vi "Holo_link_test.vi"() -> ()   [LabVIEW 2023, in "holoTracker.lvlib"]
uses:
  holoTracker.lvlib
  <vilib>/Native 3D Graph/xcontrol/3DPC_SurfacePlot.xctl
panel:
  in  "minLenght":i32
  in  "stop":bool
  out "3D Graph":refnum<class "Base Datatype.lvclass">[](xcontrol)
  out "trajectorie":dbl[][](array[numeric])
  in  "feature_number":i32
  in  "memory":i32=1
  in  "searchRange":T1={"x_range(m)"=1e-06, "y_range(m)"=1e-06, "z__range(m)"=1e-06}
  out "size(s) 3":i32[](array[numeric])=[115588, 5]
  out "size(s) 2":i32[](array[numeric])=[115588, 5]
  out "size(s)":i32[](array[numeric])=[127033, 5]
  in  "voxel_size":i32=200
  out "return value":dbl[][](array[numeric])=[[1.0, 6.084467713662889e-06, 2.7942323868046515e-05, 5.448419528875093e-07, 370.0], [1.0, 0.0001626674929866, 3.476842903182842e-05, 2.303367864442407e-06, 5232.0], [1.0, 2.1535443011089228e-05, 4.458006515051238e-05, 8.414190233452246e-06, 11468.0], [1.0, 0.0001715506368782, 4.228565376251936e-05, 5.818839099447359e-07, 292.0], [1.0, 6.632606528000906e-05, 4.749142681248486e-05, 2.467622152835247e-06, 5073.0], [1.0, 0.0001096990090445, 4.7724013711558655e-05, 1.2655297041419544e-06, 662.0], [1.0, 0.0001106120907934, 5.094841617392376e-05, 1.1342979632900096e-05, 7273.0], [1.0, 0.0001622637646505, 5.3357507567852736e-05, 1.6849965049914315e-06, 1584.0], [1.0, 0.0001665420131757, 5.386502380133607e-05, 3.075804215768585e-06, 1222.0], [1.0, 8.49634816404432e-05, 6.137051968835294e-05, 1.222071750817122e-05, 70549.0], [1.0, 0.0001014012741507, 6.489593943115324e-05, 2.9947607345093274e-06, 2263.0], [1.0, 0.0001038984846672, 7.025278318906203e-05, 2.297732862643897e-06, 1479.0], [1.0, 2.920036604336929e-05, 7.49154351069592e-05, 5.151001005287981e-06, 16448.0], [1.0, 0.000173209249624, 7.902947982074693e-05, 1.5714367691543885e-05, 11413.0], [1.0, 7.337347051361576e-05, 8.688520756550133e-05, 3.910340183210792e-06, 6218.0], [1.0, 7.923282100819051e-05, 9.101555770030244e-05, 3.967892610035051e-07, 410.0], [1.0, 6.708591536153108e-05, 9.130484977504238e-05, 3.468035458809027e-07, 397.0], [1.0, 8.80229999893345e-05, 9.468459757044911e-05, 3.539114743489336e-07, 532.0], [1.0, 6.690550071652979e-05, 9.541779581923038e-05, 3.245157529363496e-07, 254.0], [1.0, 3.5517736250767484e-05, 0.0001058862326317, 8.118919367916533e-07, 1511.0], [1.0, 2.5897679734043777e-05, 0.0001085887779481, 4.002589776064269e-06, 1483.0], [1.0, 1.948640783666633e-05, 0.000112430032459, 1.9318811155244475e-06, 3982.0], [1.0, 0.0001211502676596, 0.0001132587276515, 3.043337073904695e-06, 6890.0], [1.0, 0.0001325271732639, 0.0001166411966551, 1.7197318811668083e-05, 73988.0], [1.0, 0.0001629522594157, 0.0001161332838819, 8.296568012156058e-06, 11009.0], [1.0, 0.0001552185276523, 0.0001186439185403, 2.3219217837322503e-06, 4923.0], [1.0, 0.0001647252065595, 0.0001183489002869, 5.199617589823902e-07, 138.0], [1.0, 0.0001584361452842, 0.0001295564579777, 7.808185387148114e-07, 283.0], [1.0, 0.000158121867571, 0.0001334999979007, 8.548132655050722e-07, 581.0], [1.0, 3.150296834064648e-05, 0.0001427773095201, 2.0931878680130467e-05, 79967.0], [1.0, 1.4578064110537524e-05, 0.0001393411366734, 2.624581156851491e-06, 8022.0], [1.0, 0.000163749748026, 0.0001381954352837, 2.6074342258652905e-06, 377.0], [1.0, 7.176306826295331e-05, 0.0001397340529365, 5.237333198238048e-07, 176.0], [1.0, 0.0001668064505793, 0.0001418412430211, 3.1187559557110944e-07, 278.0], [1.0, 3.841546276817098e-05, 0.0001423163776053, 5.334248953658971e-07, 504.0], [1.0, 1.4115883459453473e-05, 0.0001550480956211, 1.0434874639031476e-05, 87692.0], [1.0, 0.0001525868719909, 0.0001566513237776, 1.6795509509393014e-05, 68919.0], [1.0, 0.0001574417838128, 0.0001585431746207, 1.4897328526330966e-07, 268.0], [1.0, 0.0001097008935175, 0.0001609185419511, 1.1331389941915404e-06, 679.0], [1.0, 0.0001519046345492, 0.000164362398209, 8.700509397385758e-07, 957.0], [1.0, 6.392512295860797e-05, 0.0001700782158877, 4.624916982720606e-06, 26125.0], [1.0, 0.0001484176609665, 0.0001732027012621, 1.917527879413683e-05, 27440.0], [1.0, 0.0001644691219553, 0.0001723233290249, 1.057493022926792e-06, 577.0], [1.0, 0.0001374908024445, 0.0001755372941261, 4.3706279484467814e-07, 430.0], [1.0, 0.0001311707601416, 0.000170940067619, 5.035582489654189e-06, 178.0], [1.0, 0.0001576331706019, 0.0001583546836627, 5.210669314692495e-06, 183.0], [1.0, 6.659836799371988e-05, 9.181829227600248e-05, 1.0223350727756042e-05, 417.0], [1.0, 0.0001582865952514, 0.0001584510609973, 1.0296550499333534e-05, 358.0], [1.0, 0.0001036058311001, 6.883801688672975e-05, 2.46377367147943e-05, 8318.0], [1.0, 0.0001612922205822, 0.0001366157957818, 2.1547250071307644e-05, 4494.0], [1.0, 0.0001656974491197, 0.0001459676132071, 1.597193295310717e-05, 1142.0], [1.0, 8.80000734468922e-05, 9.563334606355056e-05, 1.5165374861680904e-05, 155.0], [1.0, 0.0001589283929206, 0.0001584299607202, 1.4875608030706644e-05, 120.0], [1.0, 0.0001571570464875, 0.0001176301957457, 1.8592216292745437e-05, 600.0], [1.0, 9.193427831633016e-05, 0.0001520802470622, 2.448859049763996e-05, 3245.0], [1.0, 0.000112866058771, 5.088346006232314e-05, 2.0907007638015784e-05, 381.0], [1.0, 0.0001208995527122, 5.201993917580694e-05, 2.5392644602106884e-05, 4814.0], [1.0, 3.008505518664606e-05, 0.0001077202978194, 3.3227548556169495e-05, 10644.0], [1.0, 2.0109948309254836e-05, 4.9624042731011286e-05, 2.6339754185755737e-05, 1424.0], [1.0, 0.0001608280290383, 0.0001719313731882, 2.710985245357733e-05, 351.0], [1.0, 8.62869928823784e-05, 5.857026553712785e-05, 3.342138370499015e-05, 4921.0], [1.0, 0.0001626797165954, 0.0001301088195759, 3.0994753615232185e-05, 2244.0], [1.0, 4.31185144407209e-05, 7.302458834601566e-05, 3.312131957500242e-05, 3267.0], [1.0, 0.0001629685575608, 0.0001367063232464, 3.083618139498867e-05, 960.0], [1.0, 0.0001743247848935, 0.0001414648722857, 3.15434044750873e-05, 632.0], [1.0, 0.0001613891945453, 0.0001737980928737, 4.036536120111123e-05, 5237.0], [1.0, 0.0001142588298534, 7.320034637814388e-05, 4.0086662920657545e-05, 7267.0], [1.0, 9.60408360697329e-05, 3.4551776479929686e-05, 3.70402995031327e-05, 3724.0], [1.0, 9.843446605373174e-06, 0.0001594874047441, 3.914430271834135e-05, 2684.0], [1.0, 0.0001547361607663, 5.664364653057419e-05, 3.706891948240809e-05, 2573.0], [1.0, 8.177998097380623e-05, 0.0001273784146178, 4.101425656699576e-05, 5968.0], [1.0, 0.0001532866881461, 9.97651950456202e-05, 4.03202539018821e-05, 2485.0], [1.0, 8.377496851608157e-05, 6.378004036378115e-05, 4.188828825135715e-05, 2325.0], [1.0, 6.149584078229964e-05, 6.080432285671122e-05, 4.78734727948904e-05, 12097.0], [1.0, 0.0001566413993714, 2.1062844098196365e-05, 5.120203059050255e-05, 9042.0], [1.0, 7.881547207944095e-05, 8.436228381469846e-05, 4.8256984882755205e-05, 6830.0], [1.0, 9.192600373353343e-06, 0.0001562820398248, 4.230014747008681e-05, 314.0], [1.0, 3.210443537682295e-05, 0.0001058917259797, 4.397206430439837e-05, 790.0], [1.0, 1.0259605431883757e-07, 0.0001552348112454, 4.410862675285898e-05, 124.0], [1.0, 0.0001500043581472, 3.777907477342524e-05, 4.75865017506294e-05, 5899.0], [1.0, 6.773022323613986e-05, 9.073886030819268e-05, 4.405568688525818e-05, 654.0], [1.0, 7.17540315235965e-05, 9.311777830589564e-05, 4.51631894975435e-05, 120.0], [1.0, 0.0001315168628934, 0.0001169017778011, 4.3997453758493066e-05, 275.0], [1.0, 8.366083784494549e-05, 9.656340262154116e-05, 5.384273754316382e-05, 8763.0], [1.0, 0.0001212393835885, 0.0001420576445525, 4.49199287686497e-05, 319.0], [1.0, 1.3556540352510638e-06, 0.0001552532194182, 4.509215796133503e-05, 175.0], [1.0, 0.0001683209993643, 0.000177976078703, 7.403743802569807e-05, 9925.0], [1.0, 7.289469067472965e-05, 7.800028834026307e-05, 5.28059717908036e-05, 2797.0], [1.0, 6.758869858458638e-05, 9.146620141109452e-05, 5.3512281738221645e-05, 1976.0], [1.0, 7.586500578327104e-05, 0.0001471474388381, 5.1613689720397815e-05, 1663.0], [1.0, 8.421528764301911e-05, 6.580434273928404e-05, 5.2117964514764026e-05, 1109.0], [1.0, 7.542532694060355e-05, 0.0001033193984767, 5.398859138949774e-05, 1832.0], [1.0, 3.501192622934468e-05, 0.0001395642757415, 5.483976929099299e-05, 5287.0], [1.0, 4.265514508006163e-05, 0.0001677416439633, 5.720457556890324e-05, 9416.0], [1.0, 7.38311791792512e-05, 0.0001008389881462, 5.14670173288323e-05, 145.0], [1.0, 7.137070497265086e-05, 9.350352047476918e-05, 5.3323659813031554e-05, 1723.0], [1.0, 0.0001614146895008, 9.723609400680289e-05, 5.891673208680004e-05, 4327.0], [1.0, 9.978431626223028e-05, 0.0001333983673248, 5.464206333272159e-05, 396.0], [1.0, 5.090175818622811e-06, 0.0001601206022314, 5.6050434068311006e-05, 894.0], [1.0, 9.459191642235965e-05, 6.544839561684057e-05, 7.306145562324673e-05, 29371.0], [1.0, 7.746577466605231e-05, 8.46039765747264e-05, 6.175429734867066e-05, 262.0], [1.0, 0.0001582324039191, 2.1445872334879823e-05, 6.363449210766703e-05, 870.0], [1.0, 3.7317844544304535e-05, 9.124814096139744e-05, 6.831272185081616e-05, 6541.0], [1.0, 1.784480809874367e-05, 0.0001019813425955, 6.767934974050149e-05, 2458.0], [1.0, 4.959088528266875e-06, 0.0001600535470061, 8.137130498653278e-05, 29776.0], [1.0, 3.297331932117231e-05, 0.0001390695833833, 6.774533540010452e-05, 1053.0], [1.0, 8.322825306095183e-05, 0.0001434805017197, 6.561006739502773e-05, 1939.0], [1.0, 0.0001370376121485, 9.71412009675987e-06, 6.492882675956935e-05, 291.0], [1.0, 0.0001772090326994, 3.539895624271594e-05, 6.882343586767092e-05, 3231.0], [1.0, 5.806188710266724e-05, 3.3593849366297945e-05, 6.884828326292336e-05, 2367.0], [1.0, 7.016197741904762e-06, 0.0001632697239983, 6.754777859896421e-05, 243.0], [1.0, 0.000170219267602, 0.0001663451548665, 7.293584349099547e-05, 4976.0], [1.0, 2.793159910652321e-05, 0.0001489773421781, 7.33017732272856e-05, 3999.0], [1.0, 0.0001163198103313, 6.302370456978679e-05, 7.591531903017312e-05, 3997.0], [1.0, 9.778481035027652e-05, 0.0001406495284754, 7.136896601878107e-05, 522.0], [1.0, 0.0001691433571977, 5.961917963759333e-07, 8.129586058203131e-05, 4070.0], [1.0, 1.4097173334448598e-05, 8.226431236835197e-05, 7.784627086948603e-05, 6167.0], [1.0, 2.436563590890728e-05, 1.974108090507798e-05, 8.088676258921623e-05, 7748.0], [1.0, 1.164888817584142e-05, 3.0726434488315135e-05, 8.314807928400114e-05, 3895.0], [1.0, 7.282009755726904e-05, 0.0001352824474452, 7.63883363106288e-05, 4002.0], [1.0, 0.0001400399924023, 0.0001319663715548, 8.391532901441678e-05, 8537.0], [1.0, 5.5921103921718895e-05, 0.000108788088255, 9.001097350846976e-05, 17549.0], [1.0, 0.000113057278213, 6.979489990044385e-05, 9.000674617709592e-05, 13550.0], [1.0, 0.0001127664218074, 9.079198207473382e-05, 8.478527161059901e-05, 8091.0], [1.0, 5.82017055421602e-05, 0.0001726192276692, 8.456128853140399e-05, 3833.0], [1.0, 1.0619457498250997e-05, 0.0001078733839676, 8.637746941531077e-05, 2405.0], [1.0, 2.520033740438521e-05, 0.000139325245982, 8.391139999730512e-05, 213.0], [1.0, 3.813329021795653e-05, 0.0001060482827597, 9.526589565211908e-05, 7139.0], [1.0, 0.0001007989849313, 7.21739706932567e-05, 9.082954784389584e-05, 1228.0], [1.0, 2.592455712147057e-05, 0.0001495852629886, 9.255921759177e-05, 200.0], [1.0, 4.128223008592613e-05, 4.959827856509946e-05, 9.645039244787768e-05, 6037.0], [1.0, 2.4412151105934757e-05, 0.0001384778734063, 9.155422594631092e-05, 365.0], [1.0, 5.305964077706449e-05, 0.0001283856399822, 9.582766506355256e-05, 4738.0], [1.0, 6.284587288973853e-05, 0.0001460118510294, 9.61513869697228e-05, 4087.0], [1.0, 2.5871122488752007e-05, 0.0001011573331197, 9.672308078734204e-05, 6301.0], [1.0, 4.819215610041283e-05, 9.018560376716778e-05, 9.685708209872246e-05, 1391.0], [1.0, 9.311481699114664e-05, 5.986811811453663e-05, 9.666049299994484e-05, 1440.0], [1.0, 8.8207729277201e-05, 3.934404958272353e-05, 9.83873542281799e-05, 2241.0], [1.0, 9.761466935742646e-05, 6.031811426510103e-05, 9.7536867542658e-05, 136.0], [1.0, 4.385911233839579e-05, 0.0001729830109979, 9.793794743018223e-05, 170.0], [1.0, 5.7778866903390735e-05, 0.0001088508433895, 9.875508112600072e-05, 357.0]]
  in  "Frame":i32=1
  out "error out":errorcluster
  out "Features":dbl[][](array[numeric])
  in  "holo Feature file":path=path "C:/TRAVAIL/developpement/imagesHolo/1000im_manip3/HOLO_2023_06_28_11_56_10.csv"
  in  "PythonVer":string="3.10" caption="Python version"
  in  "Python/Environnement\npath":path
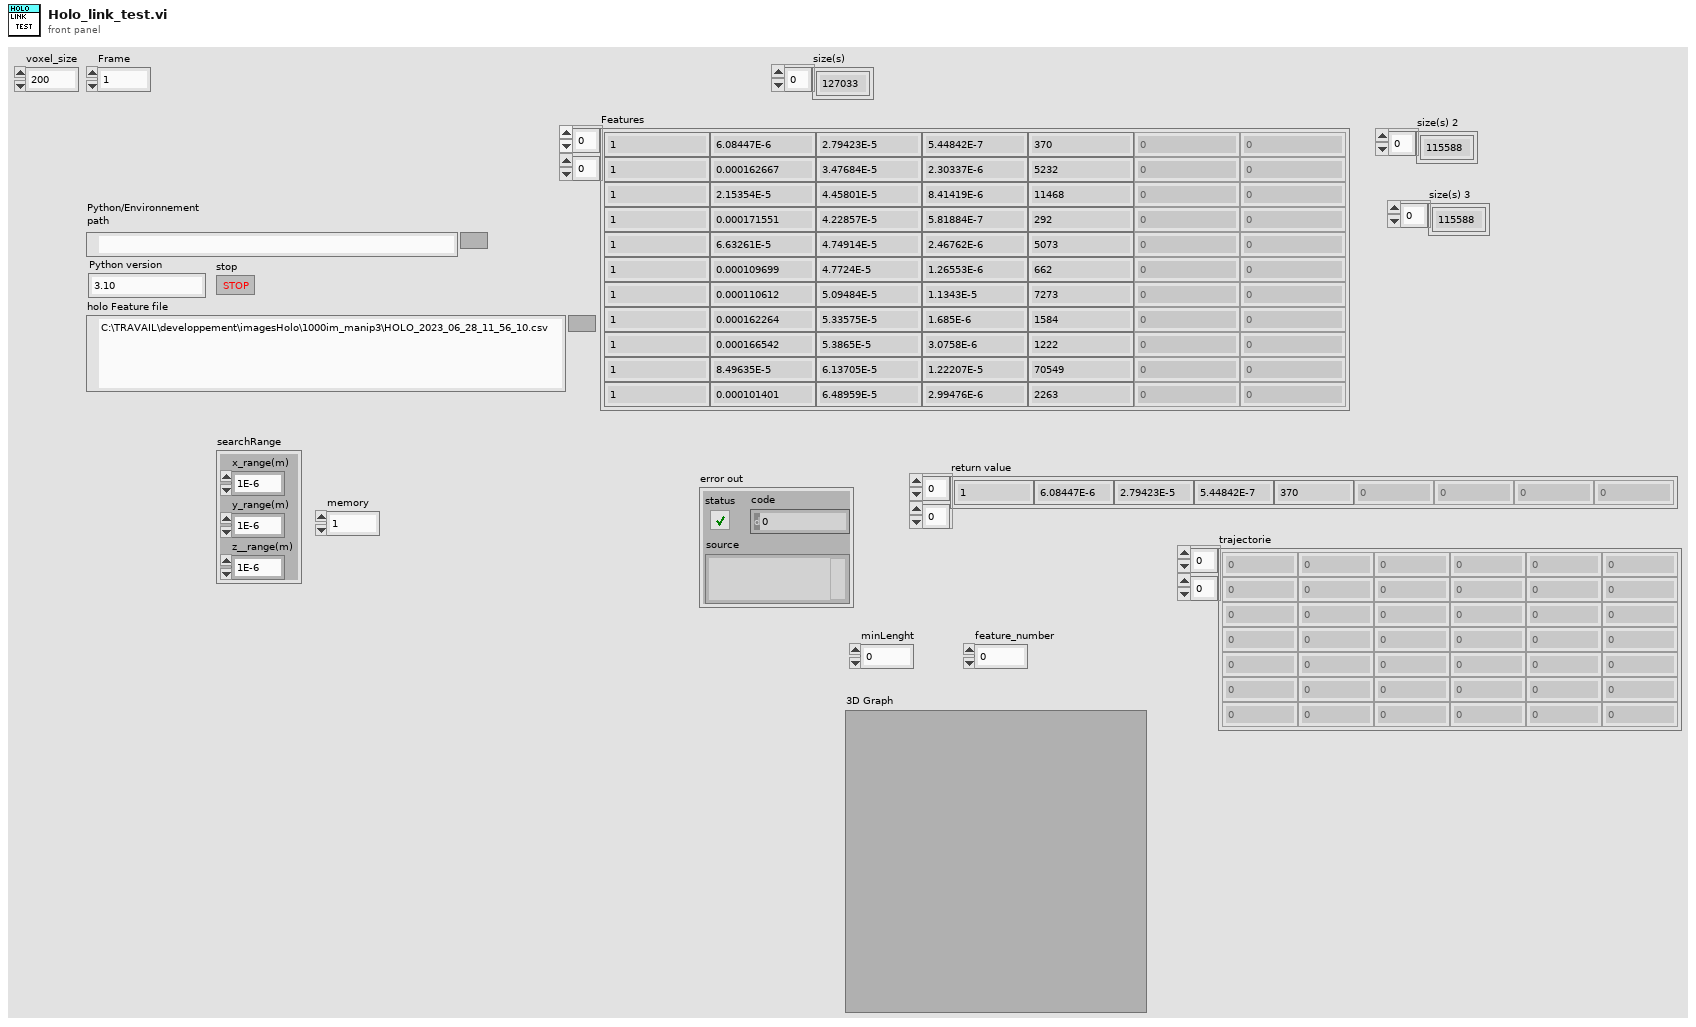
[diagram p1: front panel]
types:
  T1 = cluster{"x_range(m)":dbl, "y_range(m)":dbl, "z__range(m)":dbl}
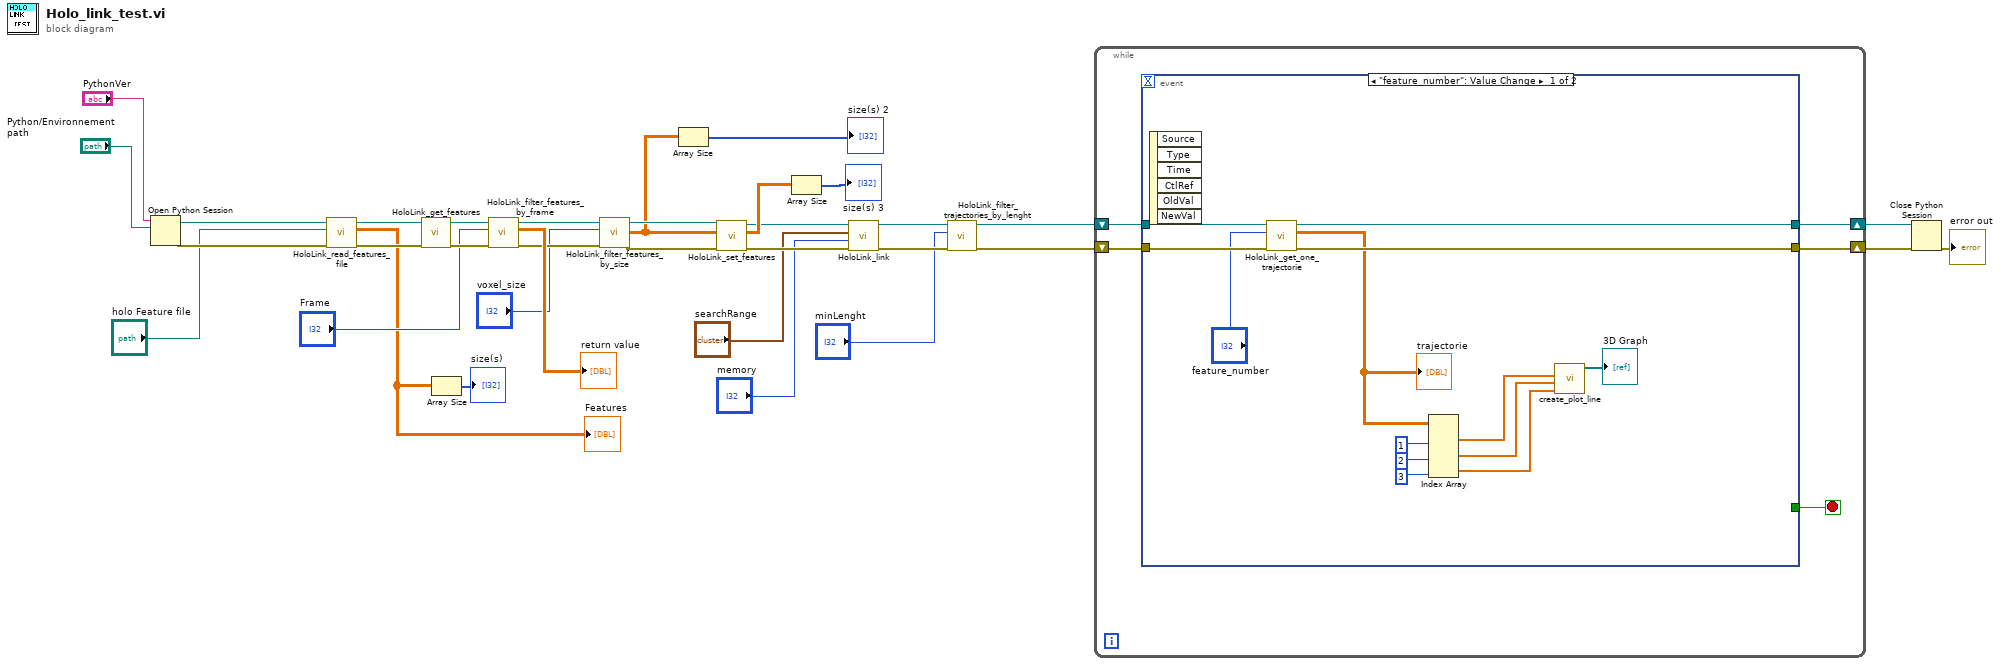
[diagram p0: block diagram]
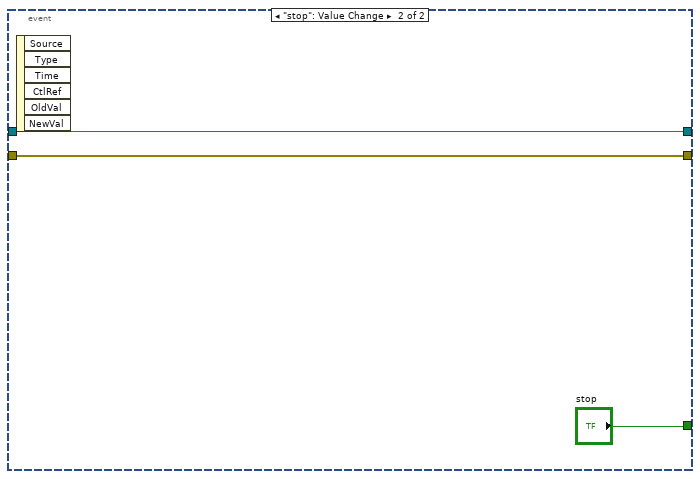
[diagram p2: hidden frame]
diagram:
  n1 = Open Python Session(python version="PythonVer", python path="Python/Environnement\npath") -> (session out=w32:refnum<k35>, error out=w31:errorcluster)  [unwired: 1 in]
  n2 = call "HoloLink_read_features_file.vi"("error in (no error)"=w31, "holo Feature file"="holo Feature file", "session in"=w32) -> ("error out"=w28:errorcluster, "localisations"=w19:dbl[][], "Refnum out"=w27:refnum<k35>)  [unwired: 6 in]
  "Features" <- w19
  n3 = call "HoloLink_get_features.vi"("error in (no error)"=w28, "session in"=w27) -> ("error out"=w25:errorcluster, "Refnum out"=w26:refnum<k35>)  [unwired: 7 in, 1 out]
  n4 = Array Size(array=w19) -> (size(s)=→"size(s)":i32[])
  n5 = call "HoloLink_filter_features_by_frame.vi"("error in (no error)"=w25, "Frame"="Frame", "session in"=w26) -> ("error out"=w21:errorcluster, "return value"=→"return value":dbl[][], "Refnum out"=w22:refnum<k35>)  [unwired: 6 in]
  n6 = call "HoloLink_filter_features_by_size.vi"("error in (no error)"=w21, "voxel_size"="voxel_size", "session in"=w22) -> ("error out"=w16:errorcluster, "return value"=w14:dbl[][], "Refnum out"=w15:refnum<k35>)  [unwired: 6 in]
  n7 = Array Size(array=w14) -> (size(s)=→"size(s) 2":i32[])
  n8 = call "HoloLink_set_features.vi"("error in (no error)"=w16, "Features"=w14, "session in"=w15) -> ("error out"=w11:errorcluster, "return value"=w12:dbl[][], "Refnum out"=w10:refnum<k35>)  [unwired: 6 in]
  n9 = Array Size(array=w12) -> (size(s)=→"size(s) 3":i32[])
  n10 = call "HoloLink_link.vi"("error in (no error)"=w11, "memory"="memory", "searchRange"="searchRange", "session in"=w10) -> ("error out"=w4:errorcluster, "Refnum out"=w5:refnum<k35>)  [unwired: 5 in, 1 out]
  n11 = call "HoloLink_filter_trajectories_by_lenght.vi"("error in (no error)"=w4, "minLenght"="minLenght", "session in"=w5) -> ("error out"=w2:errorcluster, "Refnum out"=w1:refnum<k35>)  [unwired: 6 in, 1 out]
  n12 = while {
    shift-right: [w36] -> w6
    shift-left: w1 -> [w39]
    shift-right: [w37] -> w7
    shift-left: w2 -> [w38]
    stop <- w35 stop-if-true
    n13 = event shown="[0] \"feature_number\": Value Change" {
      selector: _ -> [_ _]
      dyn-events: _ -> [_ _]
      timeout: _ -> [_ _]
      tunnel: w39 -> [w52 w54]
      tunnel: w38 -> [w51 w53]
      tunnel: [w50 w53] -> w37
      tunnel: [w49 w54] -> w36
      tunnel: [_ "stop"] -> w35
      event "feature_number": Value Change {
        n14 = event-data() -> ()  [unwired: 1 in, 6 out]
        n15 = call "HoloLink_get_one_trajectorie.vi"("error in (no error)"=w51, "feature_number"="feature_number", "session in"=w52) -> ("error out"=w50:errorcluster, "trajectorie"=w46:dbl[][], "Refnum out"=w49:refnum<k35>)  [unwired: 6 in]
        "trajectorie" <- w46
        n16 = Index Array(array=w46, index (col) #1=1 ("index (row)"), index (col) #2=2 ("index (row)"), index (col) #3=3 ("index (row)")) -> (element #1=w45:dbl[], element #2=w44:dbl[], element #3=w43:dbl[])  [unwired: 3 in]
        n17 = call <vilib>:"create_plot_line.vi"("z vector"=w43, "y vector"=w44, "x vector"=w45) -> ("plots out"=→"3D Graph":refnum<class "Base Datatype.lvclass">[])  [unwired: 2 in, 6 out]
      }
      event "stop": Value Change {
        n18 = event-data() -> ()  [unwired: 1 in, 6 out]
      }
    }
  }
  n19 = Close Python Session(session in=w6, error in=w7) -> (11:→"error out":errorcluster)
